vi "ChangeChanCurveRefDist.vi"(8 "错误输入（无错误）":errorcluster, 10 "曲线参考点距离":sgl, 11 "曲线参考点索引":u8) -> (0 "错误输出":errorcluster)   [LabVIEW 2014]
uses:
  X86Dll/ZXUTConfigMgr.dll
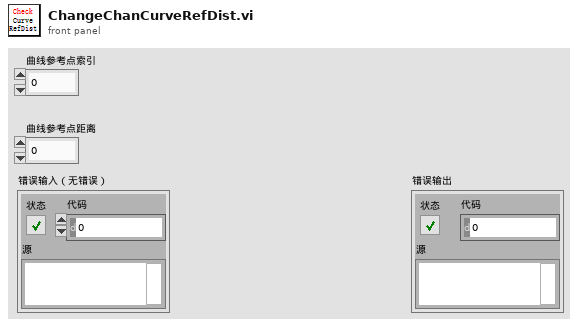
[diagram p1: front panel]
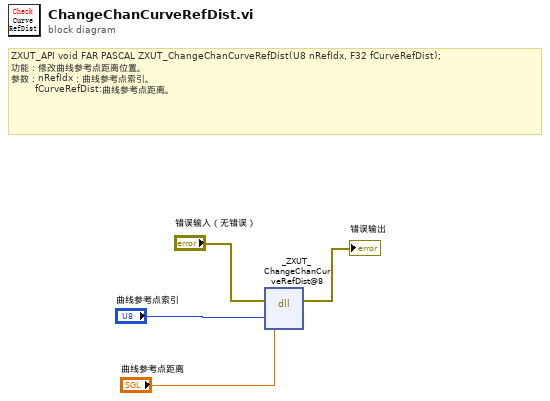
[diagram p0: block diagram]
diagram:
  # "ZXUT_API void\tFAR PASCAL ZXUT_ChangeChanCurveRefDist(U8 nRefIdx, F32 fCurveRefDist);\n功能：修改曲线参考点距离位置。\n参数：nRefIdx：曲线参考点索引。\n        fCurveRefDist:曲线参考点距离。"
  n1 = dll-call lib="D:/Software/Utrasonic on-line monitoring/X86Dll/ZXUTConfigMgr.dll" fn="_ZXUT_ChangeChanCurveRefDist@8"(error in="错误输入（无错误）", "nRefIdx"="曲线参考点索引", "fCurveRefDist"="曲线参考点距离") -> (error out=→"错误输出":errorcluster)  [unwired: 5 in, 1 out]
